vi "Read DBL.vi"(8 "error in (no error)":errorcluster, 10 "Tag":string, 11 "Var Bus in":refnum<class "Omni_Bus.lvclass">) -> (0 "error out":errorcluster, 2 "Numeric":dbl, 3 "Var Bus out":refnum<class "Omni_Bus.lvclass">)   [LabVIEW 2021, in "Omni_Bus.lvclass"]
uses:
  Omni_Bus.lvclass
  <vilib>/TSA/Abstract Data Classes/Abs_Types/Double Float/Abs_Double Float.lvclass
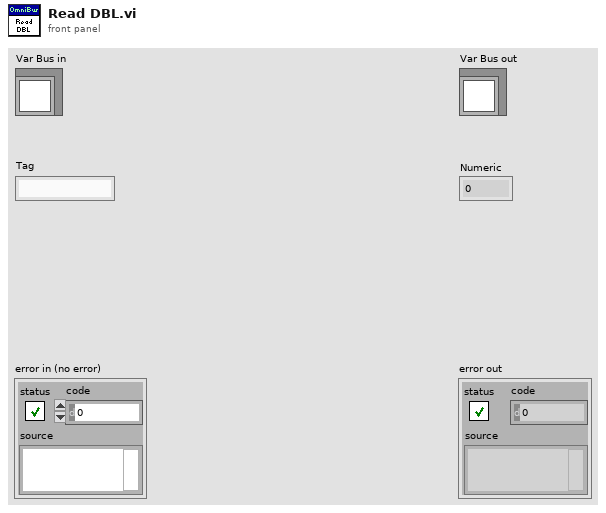
[diagram p1: front panel]
types:
  T1 = typedef "Abs_Double Float.lvclass/Type.ctl" = dbl
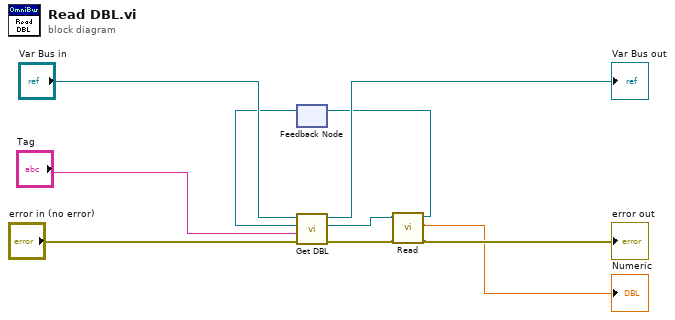
[diagram p0: block diagram]
diagram:
  n1 = feedback #1() -> (w6:refnum<class "Abs_Double Float.lvclass">)  [unwired: 1 in]
  n2 = call-dynamic "Get DBL.vi"("error in (no error)"="error in (no error)", "Tag"="Tag", "Value Type"=w6, "Var Bus in"="Var Bus in") -> ("error out"=w5:errorcluster, "Value Out"=w4:refnum<class "Abs_Double Float.lvclass">, "Var Bus out"=→"Var Bus out":refnum<class "Omni_Bus.lvclass">)  [unwired: 5 in]
  n3 = call-dynamic "Read.vi"("error in (no error)"=w5, "Double Float.lvclass_340760 in"=w4) -> ("error out"=→"error out":errorcluster, "Value"=→"Numeric":T1, "Double Float.lvclass_340760 out"=w2:refnum<class "Abs_Double Float.lvclass">)  [unwired: 7 in]
  n4 = feedback-in #1(w2) -> ()
